vi "RotatedElipse.vi"(2 "theta":dbl, 3 "Parameters":dbl[](array[numeric])) -> (0 "y out":dbl, 1 "x out":dbl)   [LabVIEW 2016]
uses:
  <vilib>/Analysis/coordinate.llb/2D Cartesian Coordinate Rotation (Scalar).vi
  <vilib>/Analysis/NI_AALPro.lvlib
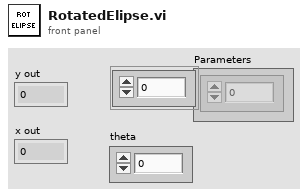
[diagram p1: front panel]
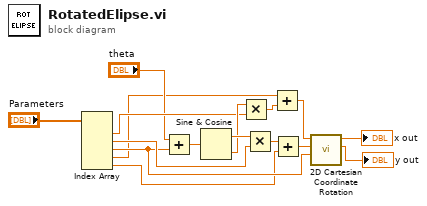
[diagram p0: block diagram]
diagram:
  n1 = Index Array(array="Parameters") -> (element #1=w13:dbl, element #2=w12:dbl, element #3=w5:dbl, element #4=w3:dbl, element #5=w1:dbl)  [unwired: 5 in]
  n2 = Add(x="theta", y=w5) -> (x+y=w6:dbl)
  n3 = Sine & Cosine(0:w6) -> (1:w16:dbl, 2:w15:dbl)
  n4 = Multiply(x=w15, y=w13) -> (x*y=w11:dbl)
  n5 = Multiply(x=w16, y=w12) -> (x*y=w10:dbl)
  n6 = Add(x=w3, y=w11) -> (x+y=w4:dbl)
  n7 = Add(x=w10, y=w1) -> (x+y=w2:dbl)
  n8 = call-poly <vilib>:"2D Cartesian Coordinate Rotation.vi"("theta"=w5, "y"=w2, "x"=w4) -> ("y out"=→"y out":dbl, "x out"=→"x out":dbl)  [unwired: 6 in, 1 out]
